vi "Ethernet TCP Read&Write.vi"(4 "Connection ID":refnum<k5>[](array[refnum]), 5 "Client?":bool, 6 "Frame Info Array":T3[](array[typedef]), 7 "Client Info":T1[](array[typedef]), 8 "error in":errorcluster, 10 "Minor Frame Freq":u8 caption="Minor Frame Time", 11 "References":T2) -> (0 "error out":errorcluster, 3 "Device Stop":bool)   [LabVIEW 2024]
doc: "All Rights Reserved © 2017 SyncSols"
uses:
  Controls/Ethernet Frame Info Cluster.ctl
  Controls/Ethernet Message Info Cluster.ctl
  Controls/Ethernet Dynamic Data Cluster.ctl
  Controls/Ethernet TCP Read Write References.ctl
  TCP Engine/Controls/TCP Engine Serial Interupt Cluster.ctl
  Controls/Ethernet Client Info Q Cluster.ctl
  Controls/Ethernet Client Info Cluster.ctl
  Controls/Ethernet Dynamic Frame Info.ctl
  TCP Engine/TCP Engine.lvlib
panel:
  out "Stop":bool=TRUE
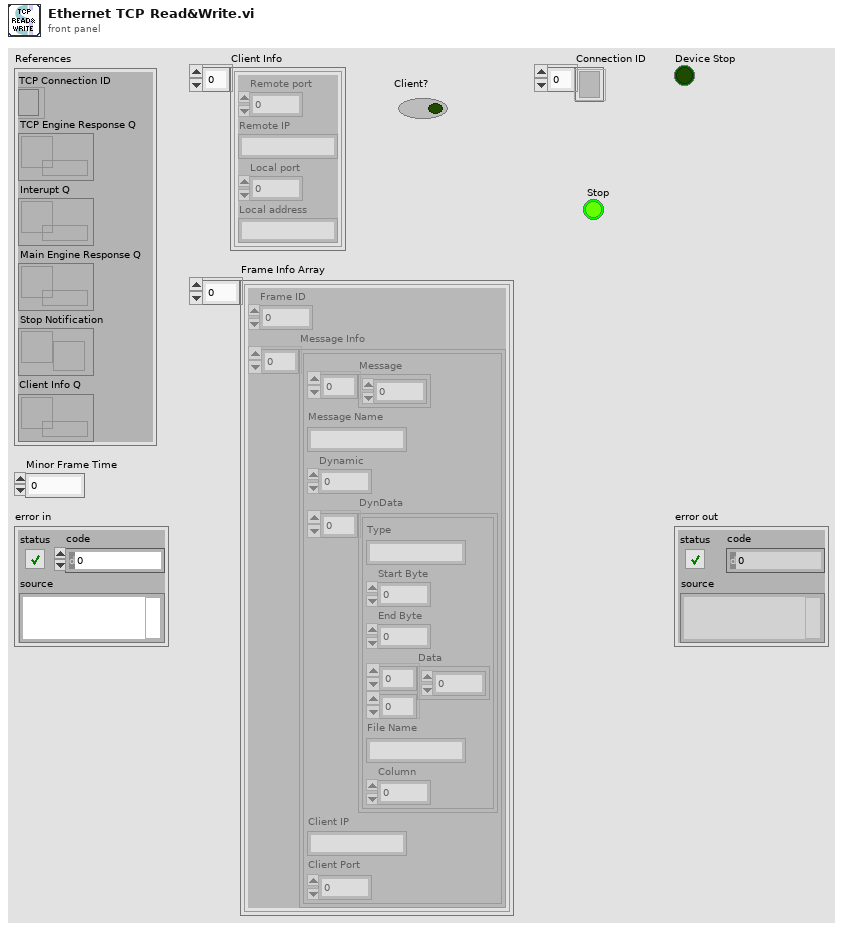
[diagram p1: front panel]
types:
  T1 = typedef "Ethernet Client Info Cluster.ctl" = cluster{"Remote port":u16, "Remote IP":string, "Local port":u16, "Local address":string}
  T2 = typedef "Ethernet TCP Read Write References.ctl" = cluster{"TCP Connection ID":refnum<k5>, "TCP Engine Response Q":refnum<queue>, "Interupt Q":refnum<queue>, "Main Engine Response Q":refnum<queue>, "Stop Notification":refnum<notifier>, "Client Info Q":refnum<queue>}
  T3 = typedef "Ethernet Frame Info Cluster.ctl" = cluster{"Frame ID":u16, "Message Info":T4[]}
  T4 = typedef "Ethernet Message Info Cluster.ctl" = cluster{"Message":u8[], "Message Name":string, "Dynamic":u8, "DynData":T5[], "Client IP":string, "Client Port":u16}
  T5 = typedef "Ethernet Dynamic Data Cluster.ctl" = cluster{"Type":string, "Start Byte":u8, "End Byte":u8, "Data":u32[][], "File Name":string, "Column":i32}
  T6 = typedef "Ethernet Dynamic Frame Info.ctl" = cluster{"Dynamic Msg Array":string[], "Dyn Column":i32[][]}
  T7 = typedef "Ethernet Client Info Q Cluster.ctl" = cluster{"TCP  ID":refnum<k5>, "Remote port":u16, "Remote IP":string}
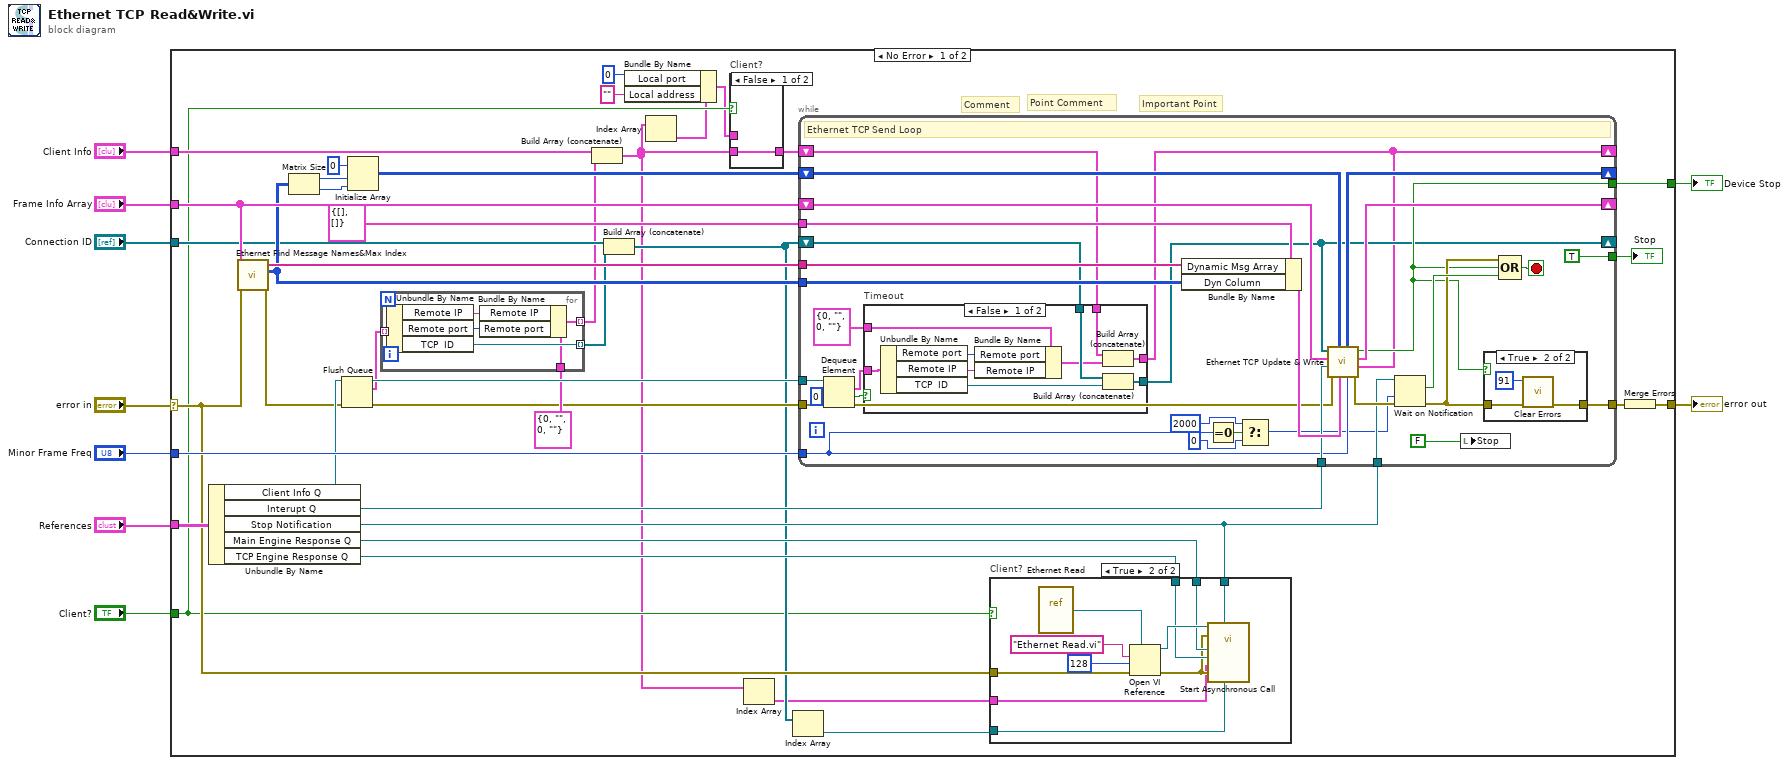
[diagram p0: block diagram]
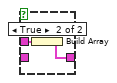
[diagram p2: hidden frame]
diagram:
  n1 = case shown="No Error" "error in" {
    selector: "error in" -> [w20 w119]
    tunnel: [w45 w119] -> w3
    tunnel: "Frame Info Array" -> [w43 _]
    tunnel: "Minor Frame Freq" -> [w47 _]
    tunnel: [w46 _] -> w6
    tunnel: "References" -> [w35 _]
    tunnel: "Connection ID" -> [w33 _]
    tunnel: "Client Info" -> [w32 _]
    tunnel: "Client?" -> [w16 _]
    frame No Error {
      # "Important Point"
      # "Point Comment"
      # "Comment"
      n2 = Unbundle By Name(w35) -> ("Client Info Q"=w31:refnum<queue>, "Interupt Q"=w34:refnum<queue>, "Stop Notification"=w22:refnum<notifier>, "Main Engine Response Q"=w23:refnum<queue>, "TCP Engine Response Q"=w24:refnum<queue>)
      n3 = call "Ethernet Find Message Names&Max Index.vi"("error in"=w20, "Frame Info"=w43) -> ("error out"=w30:errorcluster, "Dynamic column"=w37:i32[][], "Dynamic Message"=w42:string[])  [unwired: 7 in]
      n4 = Matrix Size(0:w37) -> (1:w40:i32, 2:w39:i32)
      n5 = Flush Queue(queue=w31, error in (no error)=w30) -> (queue out=w29:refnum<queue>, remaining elements=w28:T7[], error out=w21:errorcluster)
      n6 = Initialize Array(0, w40, w39) -> (w38:i32[][])
      n7 = for {
        tunnel: w28 -> [w68] mode=indexing
        tunnel: [w67] -> w25 mode=indexing
        tunnel: T1 {"Remote port"=0, "Remote IP"="", "Local port"=0, "Local address"=""} -> [w66]
        tunnel: [w63] -> w26 mode=indexing
        n8 = Unbundle By Name(w68) -> ("Remote IP"=w65:string, "Remote port"=w64:u16, "TCP  ID"=w67:refnum<k5>)
        n9 = Bundle By Name(cluster=w66, "Remote IP"=w65, "Remote port"=w64) -> (w63:T1)
      }
      n10 = Build Array (concatenate)(w32, w26) -> (w14:T1[])
      n11 = Build Array (concatenate)(w33, w25) -> (w19:refnum<k5>[])
      n12 = Index Array(array=w14) -> (element=w13:T1)  [unwired: 1 in]
      n13 = Bundle By Name(cluster=w13, "Local port"=u16 0, "Local address"="") -> (w10:T1)
      n14 = case "Client?" shown="False" w16 {
        tunnel: w14 -> [w49 _]
        tunnel: [w49 w50] -> w15
        tunnel: w10 -> [_ w51]
        frame False {
        }
        frame True {
          n15 = Build Array(w51) -> (w50:T1[])
        }
      }
      n16 = Index Array(array=w14) -> (element=w17:T1)  [unwired: 1 in]
      n17 = Index Array(array=w19) -> (element=w18:refnum<k5>)  [unwired: 1 in]
      n18 = while {
        tunnel: [w99] -> w48
        tunnel: w21 -> [w84]
        shift-right: [w98] -> _
        shift-left: w43 -> [w93]
        tunnel: w47 -> [w73]
        tunnel: [w96] -> w46
        tunnel: [TRUE] -> w44
        shift-right: [w91] -> _
        shift-left: w38 -> [w92]
        tunnel: w42 -> [w88]
        tunnel: w37 -> [w87]
        tunnel: T6 {"Dynamic Msg Array"=[], "Dyn Column"=[]} ("Dynamic Frame Info") -> [w90]
        tunnel: w34 -> [w86]
        tunnel: w22 -> [w85]
        tunnel: w29 -> [w82]
        shift-right: [w77] -> _
        shift-left: w19 -> [w78]
        shift-right: [w75] -> _
        shift-left: w15 -> [w76]
        stop <- w102 stop-if-true
        # "Ethernet TCP Send Loop"
        n19 = Dequeue Element(queue=w82, timeout in ms (-1)=0, error in (no error)=w84) -> (element=w79:T7, timed out?=w80:bool, error out=w83:errorcluster)  [unwired: 1 out]
        n20 = case "Timeout" shown="False" w80 {
          tunnel: w79 -> [w112 _]
          tunnel: [w110 w114] -> w77
          tunnel: w78 -> [w109 w114]
          tunnel: T1 {"Remote port"=0, "Remote IP"="", "Local port"=0, "Local address"=""} -> [w108 _]
          tunnel: w76 -> [w104 w113]
          tunnel: [w103 w113] -> w75
          frame False {
            n21 = Unbundle By Name(w112) -> ("Remote port"=w107:u16, "Remote IP"=w106:string, "TCP  ID"=w111:refnum<k5>)
            n22 = Bundle By Name(cluster=w108, "Remote port"=w107, "Remote IP"=w106) -> (w105:T1)
            n23 = Build Array (concatenate)(w104, w105) -> (w103:T1[])
            n24 = Build Array (concatenate)(w109, w111) -> (w110:refnum<k5>[])
          }
          frame True {
          }
        }
        n25 = Bundle By Name(cluster=w90, "Dynamic Msg Array"=w88, "Dyn Column"=w87) -> (w89:T6)
        n26 = Equal To 0?(x=w73) -> (x = 0?=w72:bool)
        n27 = Select(t=2000, s=w72, f=0 ("timeout in ms (-1)")) -> (s? t:f=w69:i32)
        n28 = call "Ethernet TCP Update & Write.vi"("Client Info"=w75, "Minor Frame Freq"=w73, "Dynamic Frame Info"=w89, "Next Index"=w92, "error in"=w83, "Interupt Q"=w86, "Frame Info Array"=w93, "Connection ID"=w77) -> ("error out"=w97:errorcluster, "Frame Info Array"=w98:T3[], "Stop"=w96:bool, "Next Index"=w91:i32[][])
        n29 = Wait on Notification(notifier=w85, timeout in ms (-1)=w69, error in (no error)=w97) -> (notification=w101:bool, error out=w100:errorcluster)  [unwired: 1 in, 2 out]
        n30 = local write "Stop"(FALSE) -> ()
        n31 = case shown="True" w96 {
          tunnel: w100 -> [w115 w118]
          tunnel: [w115 w117] -> w99
          frame False {
          }
          frame True {
            n32 = call <vilib>:"Clear Errors.vi"("error in (no error)"=w118, "specific error code to clear (0: all)"=91) -> ("error out"=w117:errorcluster)  [unwired: 4 in, 1 out]
          }
        }
        n33 = Compound Arithmetic op=OR(w100, w96, w101) -> (w102:bool)
      }
      "Stop" <- w44
      n34 = case "Client?" shown="True" w16 {
        tunnel: w24 -> [_ w58]
        tunnel: w23 -> [_ w57]
        tunnel: w22 -> [_ w56]
        tunnel: w20 -> [_ w55]
        tunnel: w18 -> [_ w53]
        tunnel: w17 -> [_ w52]
        frame False {
        }
        frame True {
          n35 = vi-ref "Ethernet Read.vi"() -> (w61:refnum<vi>)
          n36 = Open VI Reference(type specifier VI Refnum (for type only)=w61, vi path="Ethernet Read.vi", options=128, error in (no error)=w55) -> (vi reference=w62:refnum<vi>, error out=w54:errorcluster)  [unwired: 2 in]
          n37 = call-by-ref "Start Asynchronous Call"(reference=w62, error in=w54, "connection ID"=w53, "Stop Notification"=w56, "error in"=w54, "Client Info"=w52, "TCP Engine Response Q"=w58, "Main Engine Response Q"=w57) -> ()  [unwired: 5 in, 3 out]
        }
      }
      n38 = Merge Errors(w48) -> (w45:errorcluster)
    }
    frame Error {
    }
  }
  "error out" <- w3
  "Device Stop" <- w6
